vi "Config Chans Clock and Start Scanning.vi"(4 "bypass":bool, 5 "Rate":dbl=10000.0 caption="Sample Rate (Hz)" format="%0.2f", 6 "start now?":bool, 7 "sample mode":i32(ring)=10178 items=["Finite Samples"=10178, "Continuous Samples"=10123], 8 "error_in":errorcluster, 10 "SamplesPerChan":i32=1000 caption="Samples per Channel", 11 "Task in":refnum<k21>) -> (0 "error_out":errorcluster, 3 "task out":refnum<k21>)   [LabVIEW 2017]
doc: "Developed by Kevin Thompson\nThompson Engineering, LLC\nkevin@thompsonengineering.net"
uses:
  <vilib>/DAQmx/configure/timing.llb/DAQmx Timing (Sample Clock).vi
panel:
  # "Note: SamplesPerChan required if\nsample mode = \"Finite Samples\""
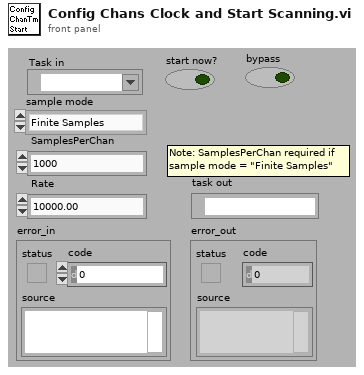
[diagram p1: front panel]
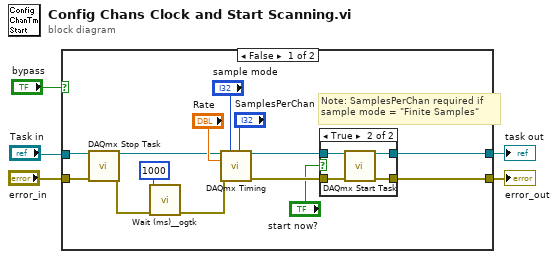
[diagram p0: block diagram]
diagram:
  n1 = case shown="False" "bypass" {
    tunnel: [w14 w26] -> w5
    tunnel: [w13 w27] -> w4
    tunnel: "error_in" -> [w11 w26]
    tunnel: "Task in" -> [w9 w27]
    frame False {
      # "Note: SamplesPerChan required if\nsample mode = \"Finite Samples\""
      n2 = call <vilib>:"DAQmx Stop Task.vi"("task/channels in"=w9, "error in"=w11) -> ("task out"=w10:refnum<k21>, "error out"=w8:errorcluster)  [unwired: 12 in]
      n3 = call <userlib>:"Wait (ms)__ogtk.vi"("error in (no error)"=w8, "milliseconds to wait"=u32 1000) -> ("error out"=w7:errorcluster)  [unwired: 8 in, 1 out]
      n4 = call-poly <vilib>:"DAQmx Timing.vi"("task/channels in"=w10, "sample mode"="sample mode", "samples per channel"="SamplesPerChan", "rate"="Rate", "error in"=w7) -> ("task out"=w15:refnum<k21>, "error out"=w16:errorcluster)  [unwired: 9 in]
      n5 = case shown="True" "start now?" {
        tunnel: w16 -> [w20 w25]
        tunnel: w15 -> [w21 w24]
        tunnel: [w20 w23] -> w14
        tunnel: [w21 w22] -> w13
        frame False {
        }
        frame True {
          n6 = call <vilib>:"DAQmx Start Task.vi"("task/channels in"=w24, "error in"=w25) -> ("task out"=w22:refnum<k21>, "error out"=w23:errorcluster)  [unwired: 12 in]
        }
      }
    }
    frame True {
    }
  }
  "error_out" <- w5
  "task out" <- w4
